vi "CloseSystemDefinitionReferences.vi"(8 "error in":errorcluster, 11 "VeriStandScriptingTestCase in":refnum<class "VeriStandScriptingTestCase.lvclass">) -> (0 "error out":errorcluster, 3 "VeriStandScriptingTestCase out":refnum<class "VeriStandScriptingTestCase.lvclass">)   [LabVIEW 2017, in "VeriStandScriptingTestCase.lvclass"]
uses:
  VeriStandScriptingTestCase.lvclass
  VeriStandScriptingTestCase.lvclass/VeriStandScriptingTestCase.ctl
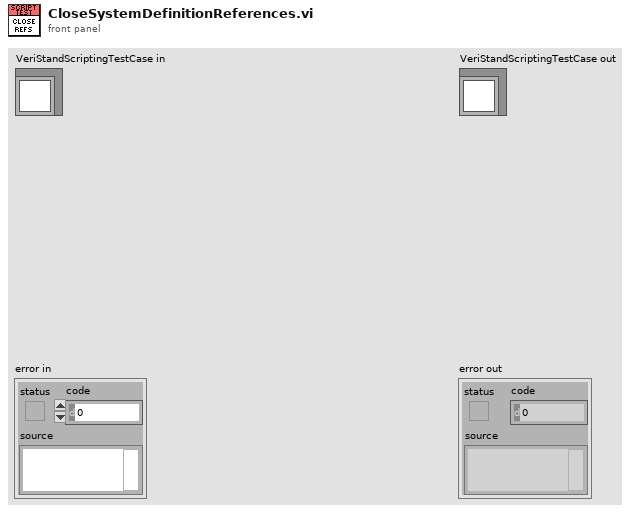
[diagram p1: front panel]
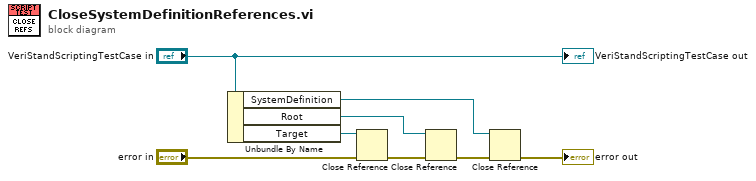
[diagram p0: block diagram]
diagram:
  n1 = Unbundle By Name("VeriStandScriptingTestCase in") -> ("SystemDefinition"=w1:refnum<k24>, "Root"=w2:refnum<k24>, "Target"=w3:refnum<k24>)
  n2 = Close Reference(reference=w3, error in (no error)="error in") -> (error out=w6:errorcluster)
  n3 = Close Reference(reference=w2, error in (no error)=w6) -> (error out=w5:errorcluster)
  n4 = Close Reference(reference=w1, error in (no error)=w5) -> (error out=→"error out":errorcluster)
  "VeriStandScriptingTestCase out" <- "VeriStandScriptingTestCase in"
